vi "Test - Thermal Chamber Controller_DQMH - Update Ramp Rate 1-setup.vi"(7 "test case ID":string, 8 "error in (no error)":errorcluster) -> (0 "error out":errorcluster, 2 "Temperature Ramp Rate":dbl format="%#_13g")   [LabVIEW 2015]
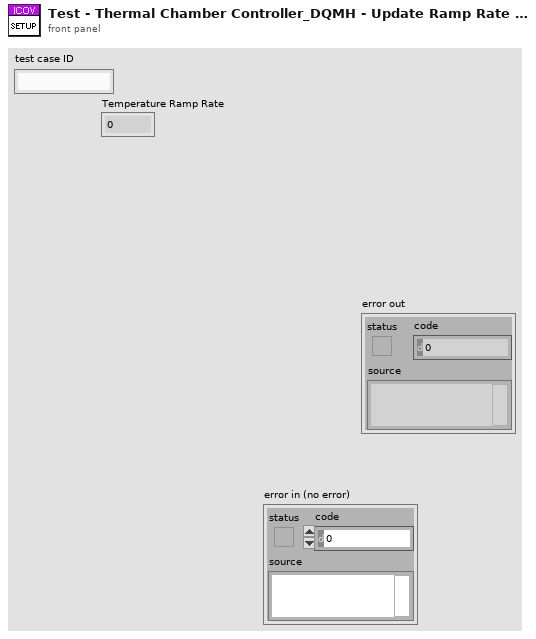
[diagram p1: front panel]
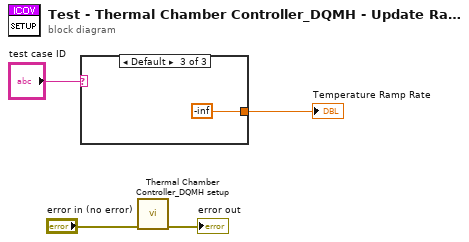
[diagram p0: block diagram]
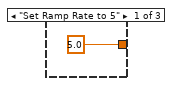
[diagram p2: hidden frame]
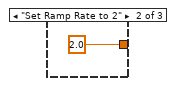
[diagram p3: hidden frame]
diagram:
  n1 = case shown="Default" "test case ID" {
    tunnel: [5.0 ("Temperature Ramp Rate 2") 2.0 ("Temperature Ramp Rate 2") -inf] -> w1
    frame "Set Ramp Rate to 5" {
    }
    frame "Set Ramp Rate to 2" {
    }
    frame Default {
    }
  }
  "Temperature Ramp Rate" <- w1
  n2 = call "Thermal Chamber Controller_DQMH setup.vi"("error in (no error)"="error in (no error)") -> ("error out"=→"error out":errorcluster)  [unwired: 10 in]
